vi "Rooted Path.vi"(11 "Path":string) -> (3 "Rooted Path":string)   [LabVIEW 2020, in "IO.lvlib" / "URI.lvclass"]
uses:
  URI.lvclass
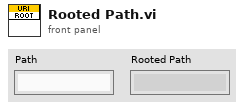
[diagram p1: front panel]
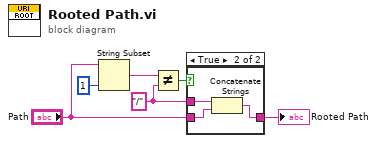
[diagram p0: block diagram]
diagram:
  w4 = "/" ("y")
  n1 = String Subset(string="Path", length (rest)=1 ("length (rest)")) -> (substring=w5:string)  [unwired: 1 in]
  n2 = Not Equal?(x=w5, y=w4) -> (x != y?=w1:bool)
  n3 = case shown="True" w1 {
    tunnel: "Path" -> [w7 w10]
    tunnel: w4 -> [_ w9]
    tunnel: [w7 w8] -> w2
    frame False {
    }
    frame True {
      n4 = Concatenate Strings(w9, w10) -> (w8:string)
    }
  }
  "Rooted Path" <- w2
